vi "libssh2_knownhost_checkp.vi"(5 "port":i32, 7 "host":string, 8 "error in (no error)":errorcluster, 9 "typemask":T3 items=["TYPE_PLAIN"=1, "TYPE_SHA1"=2, "TYPE_CUSTOM"=3, "KEYENC_RAW"=65536, "KEYENC_BASE64"=131072, "KEY_RSA1"=262144, "KEY_SSHRSA"=524288, "KEY_SSHDSS (deprecated)"=786432, "KEY_ECDSA_256"=1048576, "KEY_ECDSA_384"=1310720, "KEY_ECDSA_521"=1572864, "KEY_ED25519"=1835008, "KEY_UNKNOWN"=3932160], 10 "key":u8[](array[numeric]), 11 "host key database":T4) -> (0 "error out":errorcluster, 2 "result":T2=enum."Failure", 3 "host key":T1)   [LabVIEW 2017, in "libssh2.lvlib"]
doc: "Check if a host key is in a host key database.\n\nThis check is required before authentication. Continue only when the result is MATCH. Treat MISMATCH, NOTFOUND, and FAILURE as authentication failures."
uses:
  libssh2.lvlib
  Host Key Database Refnum.ctl
  libssh2_knownhost_typemask.ctl
  Host Key Check Result.ctl
  Host Key Refnum.ctl
  Warn Deprecated.vi
  Not A Host Key Database.vi
  <vilib>/Utility/error.llb/Error Cluster From Error Code.vi
  Global Settings.vi
  Read Host Key Database Refnum.vi
  <vilib>/Utility/semaphor.llb/Acquire Semaphore.vi
  <vilib>/Utility/semaphor.llb/Release Semaphore.vi
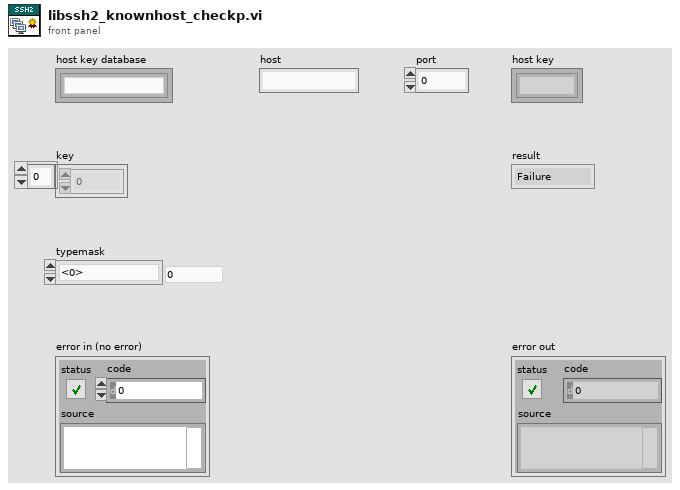
[diagram p1: front panel]
types:
  T1 = typedef "libssh2.lvlib/Host Key Refnum.ctl" = refnum<k1>
  T2 = typedef "libssh2.lvlib/Host Key Check Result.ctl" = enum16{"Match", "Mismatch", "Not Found", "Failure"}
  T3 = typedef "libssh2.lvlib/libssh2_knownhost_typemask.ctl" = i32
  T4 = typedef "libssh2.lvlib/Host Key Database Refnum.ctl" = refnum<k1>
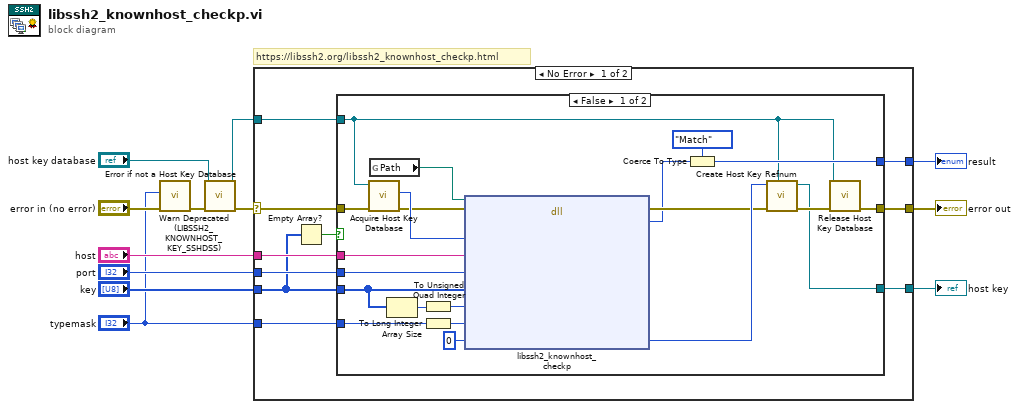
[diagram p0: block diagram]
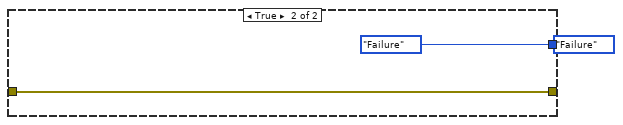
[diagram p2: hidden frame]
diagram:
  # "https://libssh2.org/libssh2_knownhost_checkp.html"
  n1 = call "Warn Deprecated (LIBSSH2_KNOWNHOST_KEY_SSHDSS).vi"("error in (no error)"="error in (no error)", "typemask"="typemask") -> ("error out"=w2:errorcluster)  [unwired: 9 in]
  n2 = call "Error if not a Host Key Database.vi"("error in (no error)"=w2, "host key database"="host key database") -> ("error out"=w6:errorcluster, "host key database out"=w4:T4)  [unwired: 8 in]
  n3 = case shown="No Error" w6 {
    selector: w6 -> [w13 w46]
    tunnel: "host" -> [w22 _]
    tunnel: "port" -> [w21 _]
    tunnel: "key" -> [w18 _]
    tunnel: "typemask" -> [w14 _]
    tunnel: [w15 _] -> w9
    tunnel: w4 -> [w17 _]
    tunnel: [w20 w46] -> w8
    tunnel: [w19 _] -> w7
    frame No Error {
      n4 = Empty Array?(array=w18) -> (empty?=w16:bool)
      n5 = case shown="False" w16 {
        tunnel: w22 -> [w43 _]
        tunnel: w21 -> [w42 _]
        tunnel: w18 -> [w41 _]
        tunnel: w14 -> [w38 _]
        tunnel: w17 -> [w23 _]
        tunnel: [w24 w45] -> w20
        tunnel: [w33 _] -> w19
        tunnel: w13 -> [w31 w45]
        tunnel: [w27 Host_Key_Check_Result."Failure" ("result")] -> w15
        frame False {
          n6 = call "Acquire Host Key Database.vi"("error in (no error)"=w31, "host key database"=w23) -> ("error out"=w36:errorcluster, "LIBSSH2_KNOWNHOSTS*"=w37:u64)  [unwired: 8 in]
          n7 = global read "Global Settings.vi" "Path"() -> (w30:path)
          n8 = Array Size(array=w41) -> (size(s)=w40:i32)
          n9 = To Unsigned Quad Integer(1:w40) -> (0:w39:u64)
          n10 = To Long Integer(number=w38) -> (32bit integer=w25:T3)
          n11 = dll-call lib="?" fn="libssh2_knownhost_checkp"(path in=w30, error in=w36, "hosts"=w37, "host"=w43, "port"=w42, "key"=w41, "keylen"=w39, "typemask"=w25, "knownhost"=u64 0) -> (error out=w32:errorcluster, "return value"=w29:i32, "knownhost"=w34:u64)  [unwired: 7 in, 1 out]
          n12 = Coerce To Type(0:w29, 1:Host_Key_Check_Result."Match" ("result")) -> (2:w27:T2)
          n13 = call "Create Host Key Refnum.vi"("host key database"=w23, "error in (no error)"=w32, "libssh2_knownhost*"=w34) -> ("error out"=w35:errorcluster, "host key"=w33:T1)  [unwired: 7 in]
          n14 = call "Release Host Key Database.vi"("error in (no error)"=w35, "host key database"=w23) -> ("error out"=w24:errorcluster)  [unwired: 9 in]
        }
        frame True {
          (unwired) Host_Key_Check_Result."Failure" ("result")
        }
      }
    }
    frame Error {
    }
  }
  "error out" <- w8
  "result" <- w9
  "host key" <- w7
